vi "State Machine Cases.vi"() -> ()   [LabVIEW 2015]
panel:
  out "Arm Set Point":dbl
  in  "Min Arm Setpoint":dbl
  in  "Max Arm Setpoint":dbl
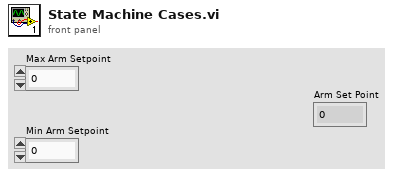
[diagram p1: front panel]
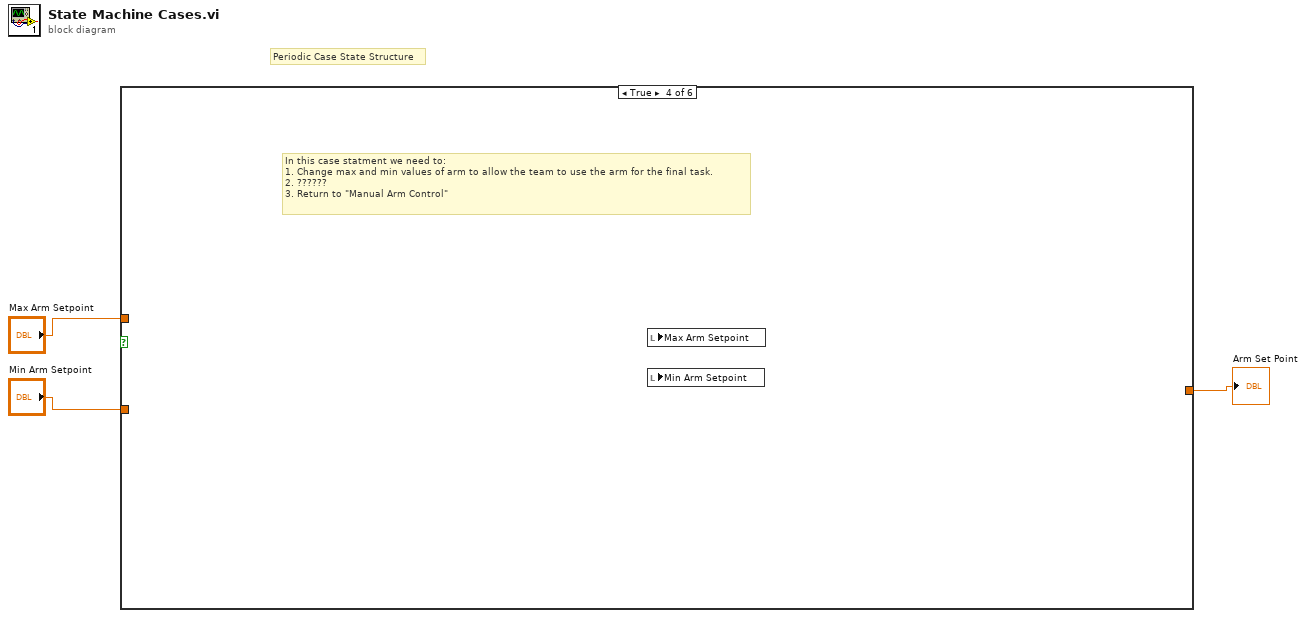
[diagram p0: block diagram]
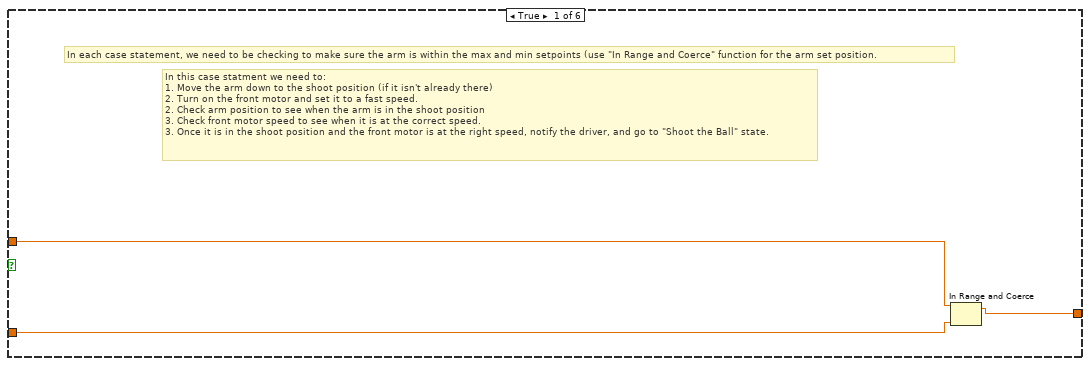
[diagram p2: hidden frame]
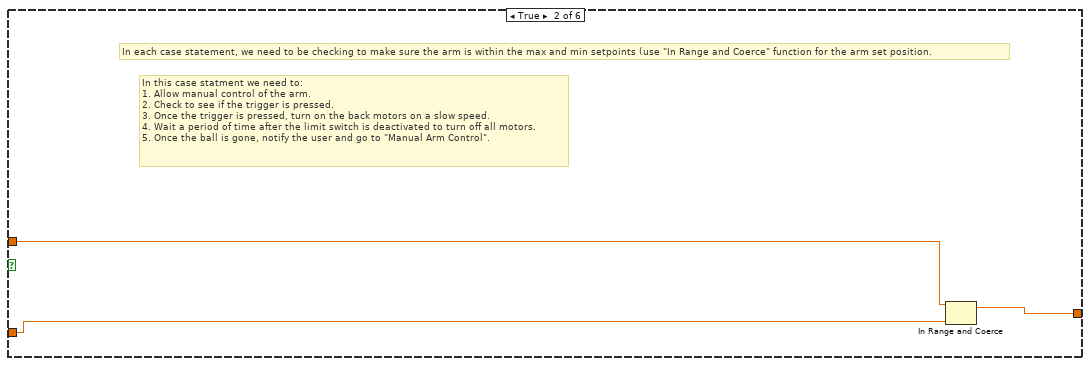
[diagram p3: hidden frame]
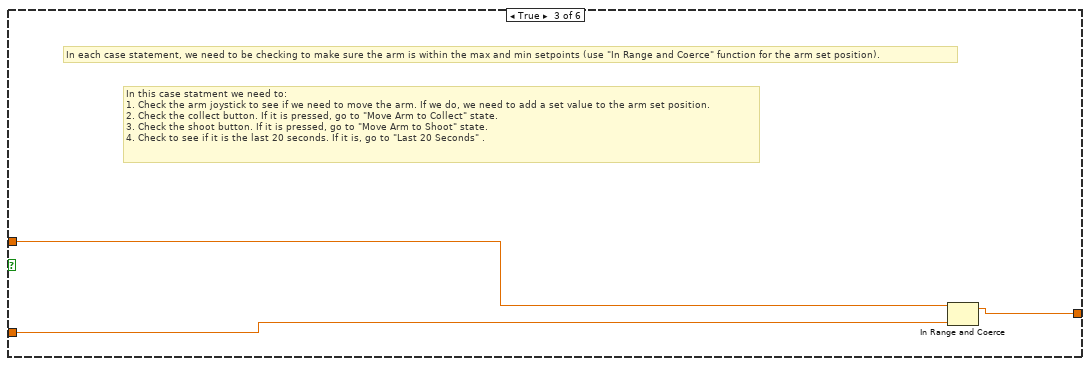
[diagram p4: hidden frame]
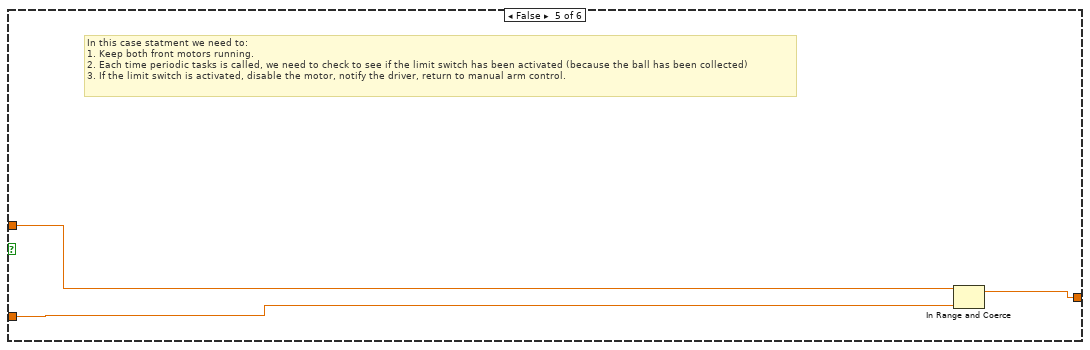
[diagram p5: hidden frame]
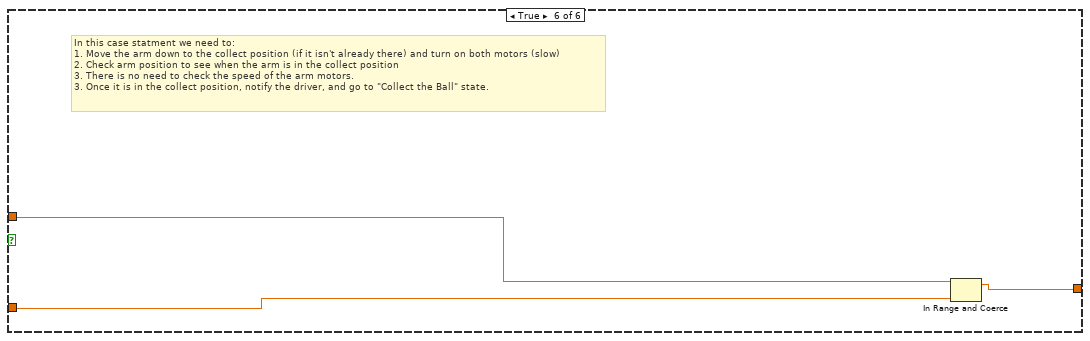
[diagram p6: hidden frame]
diagram:
  # "Periodic Case State Structure"
  n1 = case shown="\"Last 20 Seconds\"" {
    selector: _ -> [_ _ _ _ _ _]
    tunnel: "Max Arm Setpoint" -> [w6 w8 w12 _ w15 w18]
    tunnel: "Min Arm Setpoint" -> [w5 w7 w11 _ w14 w17]
    tunnel: [w4 w9 w10 _ w13 w16] -> w1
    frame True {
      # "In each case statement, we need to be checking to make sure the arm is within the max and min setpoints (use \"In Range and Coerce\" function for the arm set position."
      # "In this case statment we need to:\n1. Move the arm down to the shoot position (if it isn't already there)\n2. Turn on the front motor and set it to a fast speed.\n2. Check arm position to see when the arm is in the shoot position\n3. Check front motor speed to see when it is at the correct speed.\n3. Once it is in the shoot position and the front motor is at the right speed, notify the driver, and go to \"Shoot the Ball\" state."
      n2 = In Range and Coerce(upper limit=w6, lower limit=w5) -> (coerced(x)=w4:dbl)  [unwired: 1 in, 1 out]
    }
    frame True {
      # "In each case statement, we need to be checking to make sure the arm is within the max and min setpoints (use \"In Range and Coerce\" function for the arm set position."
      # "In this case statment we need to:\n1. Allow manual control of the arm.\n2. Check to see if the trigger is pressed.\n3. Once the trigger is pressed, turn on the back motors on a slow speed.\n4. Wait a period of time after the limit switch is deactivated to turn off all motors.\n5. Once the ball is gone, notify the user and go to \"Manual Arm Control\"."
      n3 = In Range and Coerce(upper limit=w8, lower limit=w7) -> (coerced(x)=w9:dbl)  [unwired: 1 in, 1 out]
    }
    frame True {
      # "In each case statement, we need to be checking to make sure the arm is within the max and min setpoints (use \"In Range and Coerce\" function for the arm set position)."
      # "In this case statment we need to:\n1. Check the arm joystick to see if we need to move the arm. If we do, we need to add a set value to the arm set position.\n2. Check the collect button. If it is pressed, go to \"Move Arm to Collect\" state.\n3. Check the shoot button. If it is pressed, go to \"Move Arm to Shoot\" state.\n4. Check to see if it is the last 20 seconds. If it is, go to \"Last 20 Seconds\" ."
      n4 = In Range and Coerce(upper limit=w12, lower limit=w11) -> (coerced(x)=w10:dbl)  [unwired: 1 in, 1 out]
    }
    frame True {
      # "In this case statment we need to:\n1. Change max and min values of arm to allow the team to use the arm for the final task.\n2. ??????\n3. Return to \"Manual Arm Control\""
      n5 = local read "Max Arm Setpoint"() -> ()  [unwired: 1 in]
      n6 = local read "Min Arm Setpoint"() -> ()  [unwired: 1 in]
    }
    frame False {
      # "In this case statment we need to:\n1. Keep both front motors running.\n2. Each time periodic tasks is called, we need to check to see if the limit switch has been activated (because the ball has been collected)\n3. If the limit switch is activated, disable the motor, notify the driver, return to manual arm control."
      n7 = In Range and Coerce(upper limit=w15, lower limit=w14) -> (coerced(x)=w13:dbl)  [unwired: 1 in, 1 out]
    }
    frame True {
      # "In this case statment we need to:\n1. Move the arm down to the collect position (if it isn't already there) and turn on both motors (slow)\n2. Check arm position to see when the arm is in the collect position\n3. There is no need to check the speed of the arm motors.\n3. Once it is in the collect position, notify the driver, and go to \"Collect the Ball\" state."
      n8 = In Range and Coerce(upper limit=w18, lower limit=w17) -> (coerced(x)=w16:dbl)  [unwired: 1 in, 1 out]
    }
  }
  "Arm Set Point" <- w1
